vi "Horizontal Field of View Experiment.vi"() -> ()   [LabVIEW 2019]
panel:
  out "Error (%)":dbl[](array[numeric]) format="%.1f"
  out "Actual Angle":dbl[](array[numeric]) format="%.1f"
  out "Estimated Angle":dbl[](array[numeric]) format="%.1f"
  out "XY Graph":T1(graph)
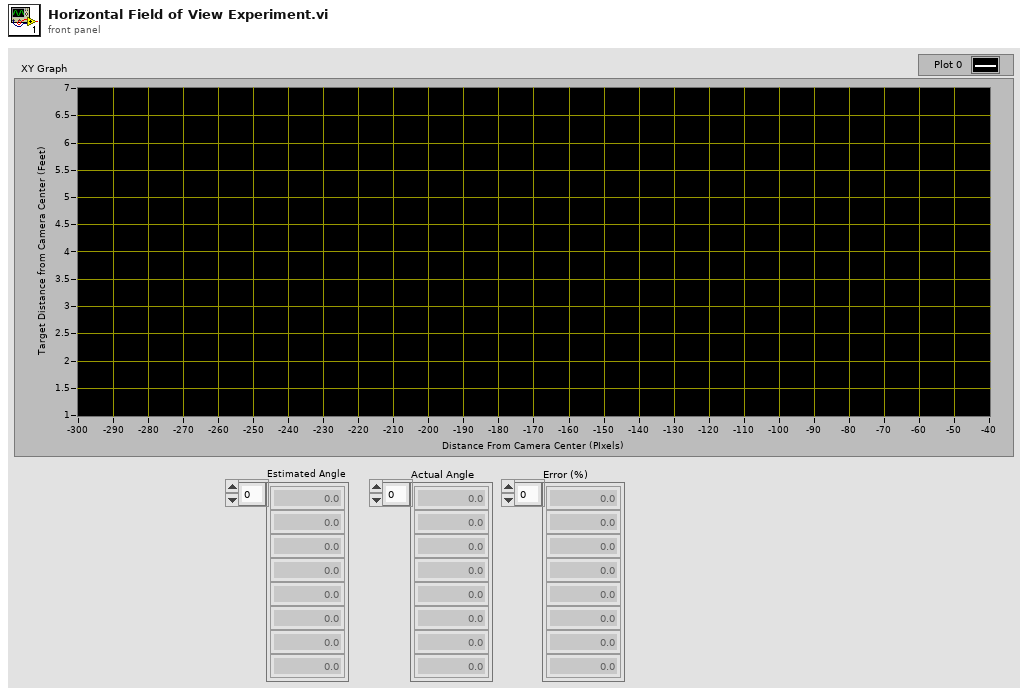
[diagram p1: front panel]
types:
  T1 = cluster{"Pixel Value":dbl[], "Feet From Center of Image":dbl[]}
  T2 = cluster{dbl[], "Feet From Center of Image":dbl[]}
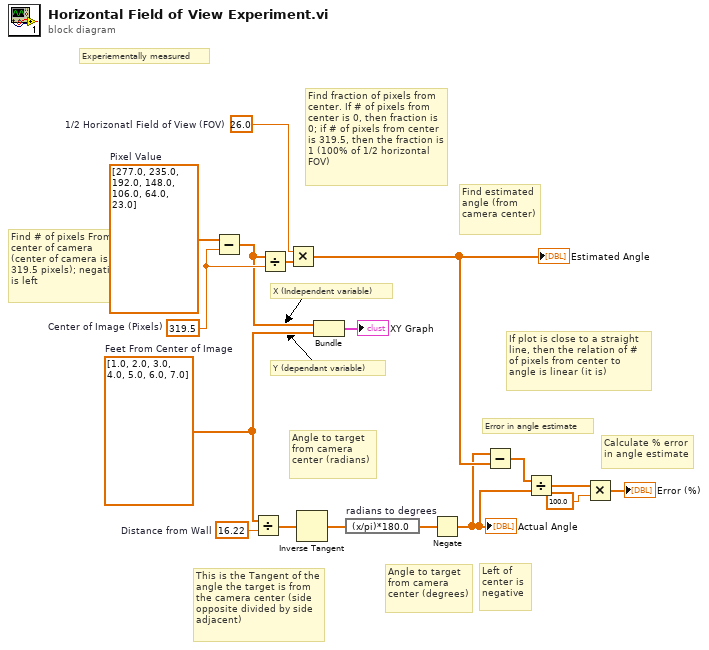
[diagram p0: block diagram]
diagram:
  w9 = 26.0  # 1/2 Horizonatl Field of View (FOV)
  w14 = 16.22  # Distance from Wall
  w11 = 319.5  # Center of Image (Pixels)
  w16 = dbl[] [277.0, 235.0, 192.0, 148.0, 106.0, 64.0, 23.0]  # Pixel Value
  w15 = dbl[] [1.0, 2.0, 3.0, 4.0, 5.0, 6.0, 7.0]  # Feet From Center of Image
  # "Calculate % error in angle estimate"
  # "Error in angle estimate"
  # "Left of center is negative"
  # "Angle to target from camera center (degrees)"
  # "Angle to target from camera center (radians)"
  # "This is the Tangent of the angle the target is from the camera center (side opposite divided by side adjacent)"
  # "Find estimated angle (from camera center)"
  # "Find fraction of pixels from center. If # of pixels from center is 0, then fraction is 0; if # of pixels from center is 319.5, then the fraction is 1 (100% of 1/2 horizontal FOV)"
  # "Experiementally measured"
  # "Find # of pixels From center of camera (center of camera is 319.5 pixels); negative is left"
  # "If plot is close to a straight line, then the relation of # of pixels from center to angle is linear (it is)"
  # "Y (dependant variable)"
  # "X (Independent variable)"
  n1 = Subtract(x=w16, y=w11) -> (x-y=w7:dbl[])
  n2 = Divide(x=w15, y=w14) -> (x/y=w13:dbl[])
  n3 = Divide(x=w7, y=w11) -> (x/y=w10:dbl[])
  n4 = Multiply(x=w9, y=w10) -> (x*y=w6:dbl[])
  "Estimated Angle" <- w6
  n5 = Inverse Tangent(1:w13) -> (0:w12:dbl[])
  n6 = Bundle(w7, "Feet From Center of Image"=w15) -> (→"XY Graph":T2)  [unwired: 1 in]
  n7 = expression code="(x/pi)*180.0" "radians to degrees"(w12) -> (w8:dbl[])
  n8 = Negate(x=w8) -> (-x=w5:dbl[])
  "Actual Angle" <- w5
  n9 = Subtract(x=w5, y=w6) -> (x-y=w2:dbl[])
  n10 = Divide(x=w2, y=w5) -> (x/y=w3:dbl[])
  n11 = Multiply(x=w3, y=100.0) -> (x*y=→"Error (%)":dbl[])
